vi "soundwave_generator_v02_file_generator_no_clicks.vi"() -> ()   [LabVIEW 2019]
uses:
  <vilib>/sound2/lvsound2.llb/Sampling Mode.ctl
  <vilib>/sound2/lvsound2.llb/Sound Data Format.ctl
  <vilib>/sound2/lvsound2.llb/Sound File Write Open.vi
  <vilib>/Waveform/WDTOps.llb/WDT Waveform Duration DBL.vi
  <vilib>/sound2/lvsound2.llb/Sound File Write (DBL).vi
  <vilib>/sound2/lvsound2.llb/Sound Output Set Volume (Single).vi
  <vilib>/sound2/lvsound2.llb/Sound Output Write (DBL).vi
  <vilib>/measure/NI_MABase.lvlib
panel:
  in  "sample duration [s]":dbl=3.0 min=0.0
  in  "File Path Control":path=path "D:/Scuola Superiore Sant'Anna/Neuro-Robotic Touch Laboratory - PhD Marian Statache - PhD Marian Statache/03 - HW & SW/Sound Psychophysical Protocol v3/sound_samples/test.wav"
  in  "frequency 2 [Hz]":dbl=43.98 min=0.0
  in  "frequency 1 [Hz]":dbl=41.28 min=0.0
  in  "Volume":dbl(slide)=50.0 min=0.0 max=100.0 step=1.0 scale=0.0..100.0
  in  "OK Button":bool
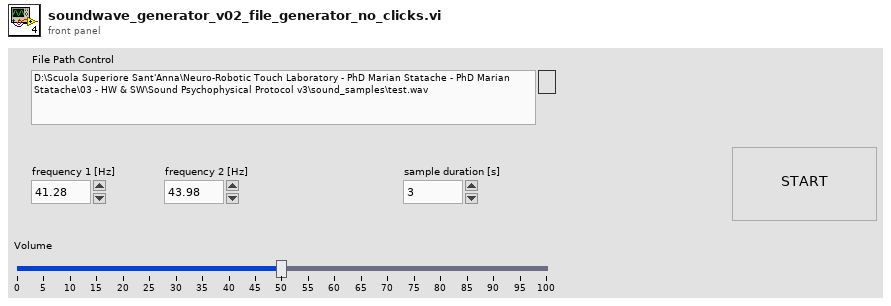
[diagram p1: front panel]
types:
  T1 = typedef "Sound Data Format.ctl" = cluster{"sample rate (S/s)":dbl, "number of channels":i32, "bits per sample":i32}
  T2 = typedef "Sampling Mode.ctl" = i32
  T3 = typedef "Sound File Refnum.ctl" = refnum<file>
  T4 = typedef "Sound Output Task ID.ctl" = u32
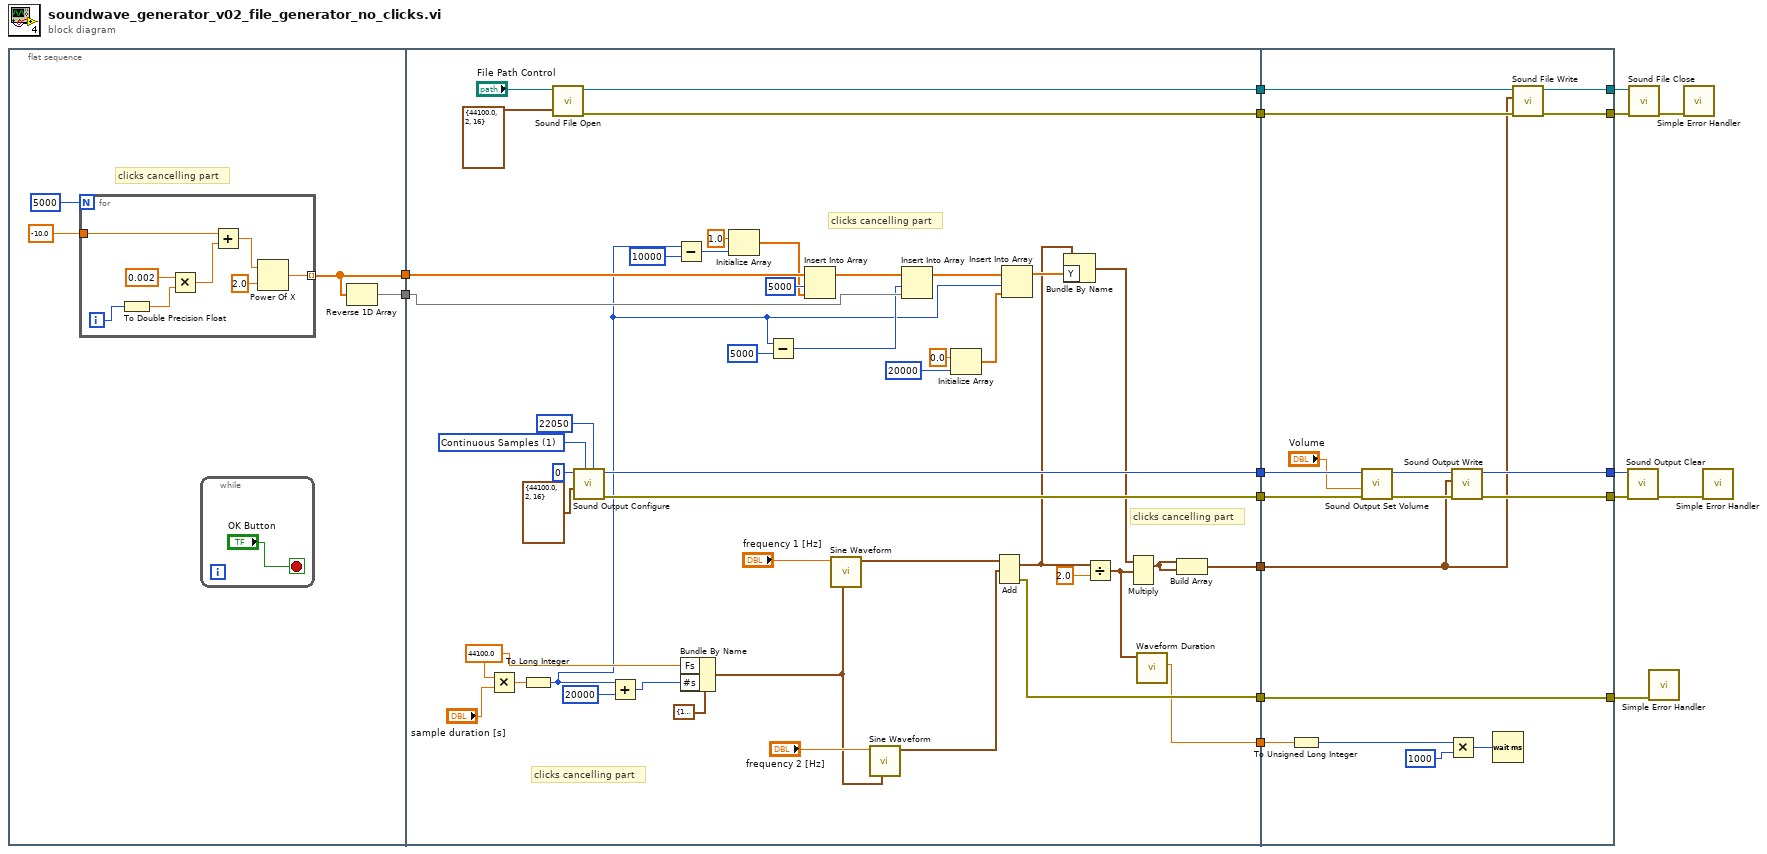
[diagram p0: block diagram]
diagram:
  n1 = flat-sequence {
    tunnel: [w17] -> w2
    tunnel: [w18] -> w1
    tunnel: [w74] -> w16
    tunnel: [w73] -> w15
    tunnel: [w72] -> w11
    tunnel: [w71] -> w10
    tunnel: [w62] -> w6
    tunnel: [w65] -> w5
    tunnel: [w63] -> w3
    tunnel: w2 -> [w43]
    tunnel: w1 -> [w48]
    tunnel: w16 -> [w91]
    tunnel: w15 -> [w90]
    tunnel: [w89] -> w14
    tunnel: [w88] -> w13
    tunnel: w11 -> [w87]
    tunnel: w10 -> [w86]
    tunnel: [w85] -> w9
    tunnel: [w84] -> w8
    tunnel: w6 -> [w80]
    tunnel: [w79] -> w4
    tunnel: w5 -> [w79]
    tunnel: w3 -> [w76]
    frame #0 {
      # "clicks cancelling part"
      n2 = for {
        N: 5000 -> [_]
        tunnel: -10.0 -> [w28]
        tunnel: [w21] -> w18 mode=indexing
        i -> [w25]
        n3 = To Double Precision Float(number=w25) -> (double precision float=w24:dbl)
        n4 = Multiply(x=0.002, y=w24) -> (x*y=w27:dbl)
        n5 = Add(x=w28, y=w27) -> (x+y=w23:dbl)
        n6 = Power Of X(1:2.0 ("x"), 2:w23) -> (0:w21:dbl)
      }
      n7 = while {
        stop <- "OK Button" stop-if-true
      }
      n8 = Reverse 1D Array(array=w18) -> (reversed array=w17:dbl[])
    }
    frame #1 {
      w55 = 44100.0 ("x")
      w61 = T2 1 items=["Finite Samples", "Continuous Samples"] ("sample mode")
      # "clicks cancelling part"
      # "clicks cancelling part"
      # "clicks cancelling part"
      n9 = Multiply(x=w55, y="sample duration [s]") -> (x*y=w56:dbl)
      n10 = To Long Integer(number=w56) -> (32bit integer=w37:i32)
      n11 = call-poly <vilib>:"Sound File Open.vi"("sound format"=T1 {"sample rate (S/s)"=44100.0, "number of channels"=2, "bits per sample"=16}, "path"="File Path Control") -> ("error out"=w71:errorcluster, "sound file refnum"=w72:T3)  [unwired: 8 in]
      n12 = call <vilib>:"Sound Output Configure.vi"("number of samples/ch"=22050, "sample mode"=w61, "sound format"=T1 {"sample rate (S/s)"=44100.0, "number of channels"=2, "bits per sample"=16}, "device ID"=u32 0) -> ("error out"=w74:errorcluster, "task ID"=w73:T4)  [unwired: 6 in]
      n13 = Add(x=w37, y=20000) -> (x+y=w50:i32)
      n14 = Subtract(x=w37, y=10000) -> (x-y=w45:i32)
      n15 = Bundle By Name(cluster=cluster{"Fs":dbl, "#s":dbl} {"Fs"=1000.0, "#s"=1000.0} ("sampling info"), "Fs"=w55, "#s"=w50) -> (w64:cluster{"Fs":dbl, "#s":dbl})
      n16 = Initialize Array(1.0 ("element"), w45) -> (w35:dbl[])
      n17 = Subtract(x=w37, y=5000) -> (x-y=w41:i32)
      n18 = Insert Into Array(array=w48, index=5000, new element=w35) -> (w44:dbl[])
      n19 = call <vilib>:"Sine Waveform.vi"("sampling info"=w64, "frequency"="frequency 1 [Hz]") -> ("signal out"=w66:waveform(dbl))  [unwired: 8 in, 1 out]
      n20 = call <vilib>:"Sine Waveform.vi"("sampling info"=w64, "frequency"="frequency 2 [Hz]") -> ("signal out"=w67:waveform(dbl))  [unwired: 8 in, 1 out]
      n21 = Insert Into Array(array=w44, index=w41, new element=w43) -> (w36:dbl[])
      n22 = Initialize Array(0.0 ("element"), 20000 ("dimension size")) -> (w38:dbl[])
      n23 = Add(1:w67, 2:w66) -> (0:w30:waveform(dbl), 3:w65:errorcluster)  [unwired: 1 in]
      n24 = Insert Into Array(array=w36, index=w37, new element=w38) -> (w34:dbl[])
      n25 = Bundle By Name(cluster=w30, "Y"=w34) -> (w33:waveform(dbl))
      n26 = Divide(x=w30, y=2.0) -> (x/y=w32:waveform(dbl))
      n27 = Multiply(1:w32, 2:w33) -> (0:w31:waveform(dbl))  [unwired: 1 in, 1 out]
      n28 = call-poly <vilib>:"Waveform Duration.vi"("waveform in"=w32) -> ("duration"=w63:dbl)  [unwired: 8 in, 2 out]
      n29 = Build Array(w31, w31) -> (w62:waveform(dbl)[])
    }
    frame #2 {
      n30 = To Unsigned Long Integer(number=w76) -> (unsigned 32bit integer=w75:u32)
      n31 = call-poly <vilib>:"Sound Output Set Volume.vi"("error in (no error)"=w91, "volume"="Volume", "task ID"=w90) -> ("error out"=w81:errorcluster, "task ID out"=w82:T4)  [unwired: 7 in]
      n32 = Multiply(x=w75, y=u32 1000) -> (x*y=w77:u32)
      n33 = call-poly <vilib>:"Sound Output Write.vi"("error in (no error)"=w81, "data"=w80, "task ID"=w82) -> ("error out"=w89:errorcluster, "task ID out"=w88:T4)  [unwired: 7 in]
      n34 = Wait (ms)(milliseconds to wait=w77) -> ()  [unwired: 1 out]
      n35 = call-poly <vilib>:"Sound File Write.vi"("error in (no error)"=w86, "data"=w80, "sound file refnum"=w87) -> ("error out"=w84:errorcluster, "sound file refnum out"=w85:T3)  [unwired: 7 in]
    }
  }
  n36 = call <vilib>:"Sound Output Clear.vi"("error in (no error)"=w14, "task ID"=w13) -> ("error out"=w12:errorcluster)  [unwired: 9 in]
  n37 = call <vilib>:"Sound File Close.vi"("error in (no error)"=w8, "sound file refnum"=w9) -> ("error out"=w7:errorcluster)  [unwired: 9 in]
  n38 = call <vilib>:"Simple Error Handler.vi"("error in (no error)"=w4) -> ()  [unwired: 4 in, 5 out]
  n39 = call <vilib>:"Simple Error Handler.vi"("error in (no error)"=w7) -> ()  [unwired: 4 in, 5 out]
  n40 = call <vilib>:"Simple Error Handler.vi"("error in (no error)"=w12) -> ()  [unwired: 4 in, 5 out]
